vi "(SubVI)Calculate DNA geometry of Length and Force.vi"(5 "Force constant (pN/nm)":dbl=0.0154, 6 "trap height(nm)":dbl, 7 "bead radius(nm)":dbl=515.0, 8 "Focal shift factor":dbl=1.22, 10 "Xst":dbl[](array[numeric]), 11 "Xbd":dbl[](array[numeric])) -> (0 "zbd (nm)":dbl[](array[numeric]), 2 "xDNA":dbl[](array[numeric]), 3 "Force":dbl[](array[numeric]))   [LabVIEW 2014]
panel:
  in  "kx/kz":dbl=3.6
  out "Fx":dbl
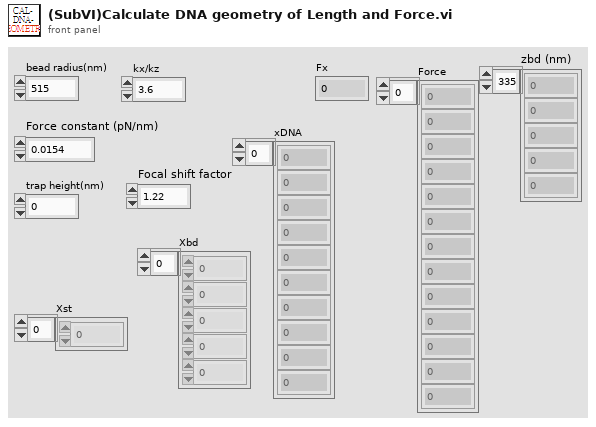
[diagram p1: front panel]
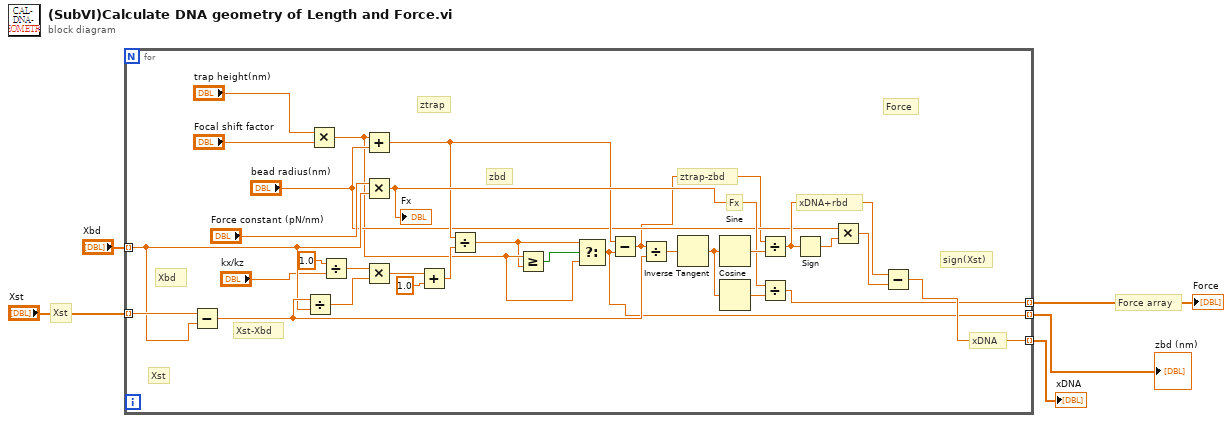
[diagram p0: block diagram]
diagram:
  # "Force array"
  # "Xst"
  n1 = for {
    tunnel: "Xst" -> [w24] mode=indexing
    tunnel: "Xbd" -> [w19] mode=indexing
    tunnel: [w23] -> w4 mode=indexing
    tunnel: [w22] -> w5 mode=indexing
    tunnel: [w6] -> w1 mode=indexing
    # "ztrap"
    # "xDNA"
    # "xDNA+rbd"
    # "Force"
    # "Fx"
    # "sign(Xst)"
    # "ztrap-zbd"
    # "Xst-Xbd"
    # "zbd"
    # "Xst"
    # "Xbd"
    n2 = Subtract(x=w24, y=w19) -> (x-y=w31:dbl)
    n3 = Divide(x=w31, y=w19) -> (x/y=w35:dbl)
    n4 = Multiply(x="trap height(nm)", y="Focal shift factor") -> (x*y=w8:dbl)
    n5 = Divide(x=1.0, y="kx/kz") -> (x/y=w16:dbl)
    n6 = Add(x=w8, y="bead radius(nm)") -> (x+y=w12:dbl)
    n7 = Multiply(x="Force constant (pN/nm)", y=w19) -> (x*y=w18:dbl)
    "Fx" <- w18
    n8 = Multiply(x=w16, y=w35) -> (x*y=w33:dbl)
    n9 = Add(x=w33, y=1.0) -> (x+y=w32:dbl)
    n10 = Divide(x=w12, y=w32) -> (x/y=w7:dbl)
    n11 = Greater Or Equal?(x=w8, y=w7) -> (x >= y?=w11:bool)
    n12 = Select(t=w7, s=w11, f=w8) -> (s? t:f=w6:dbl)
    n13 = Subtract(x=w12, y=w6) -> (x-y=w9:dbl)
    n14 = Divide(x=w9, y=w31) -> (x/y=w30:dbl)
    n15 = Inverse Tangent(1:w30) -> (0:w28:dbl)
    n16 = Sine(x=w28) -> (sin(x)=w29:dbl)
    n17 = Cosine(x=w28) -> (cos(x)=w27:dbl)
    n18 = Divide(x=w9, y=w29) -> (x/y=w21:dbl)
    n19 = Divide(x=w18, y=w27) -> (x/y=w22:dbl)
    n20 = Sign(1:w21) -> (0:w26:dbl)
    n21 = Multiply(x="bead radius(nm)", y=w26) -> (x*y=w25:dbl)
    n22 = Subtract(x=w21, y=w25) -> (x-y=w23:dbl)
  }
  "Force" <- w5
  "xDNA" <- w4
  "zbd (nm)" <- w1
